vi "encode string.vi"(11 "String":string) -> (3 "byte array out":u8[](array[numeric]))   [LabVIEW 2013, in "protocol buffers encoder.lvlib"]
uses:
  protocol buffers encoder.lvlib
panel:
  out "mgerr":i32
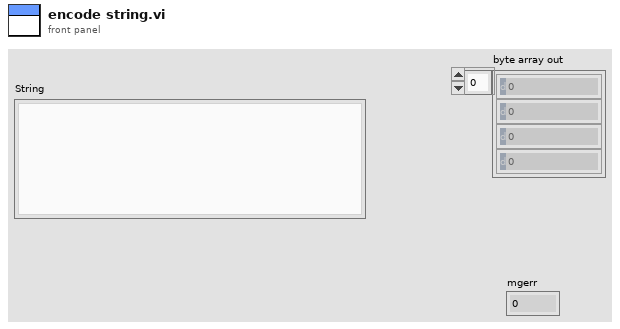
[diagram p1: front panel]
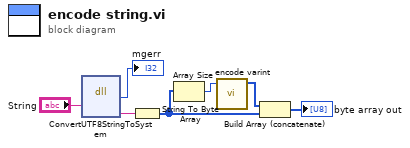
[diagram p0: block diagram]
diagram:
  n1 = dll-call lib="LabVIEW" fn="ConvertUTF8StringToSystem"("input"="String") -> ("mgerr"=→"mgerr":i32, "output"=w6:string)  [unwired: 5 in, 2 out]
  n2 = String To Byte Array(string=w6) -> (unsigned byte array=w4:u8[])
  n3 = Array Size(array=w4) -> (size(s)=w1:i32)
  n4 = call "encode varint.vi"("value"=w1) -> ("byte array out"=w5:u8[])  [unwired: 10 in]
  n5 = Build Array (concatenate)(w5, w4) -> (→"byte array out":u8[])
